vi "SetSettings.vi"(8 "error in (no error)":errorcluster, 10 "Variant":variant, 11 "NHRDCPower in":refnum<class "NHRDCPower.lvclass">) -> (0 "error out":errorcluster, 3 "NHRDCPower Out":refnum<class "NHRDCPower.lvclass">)   [LabVIEW 2018, in "AcPwrPlugins.lvlib" / "NHRDCPower.lvclass"]
doc: "This VI sets the configuration settings, measurement settings, and measurement refresh time."
uses:
  NHRDCPower.lvclass
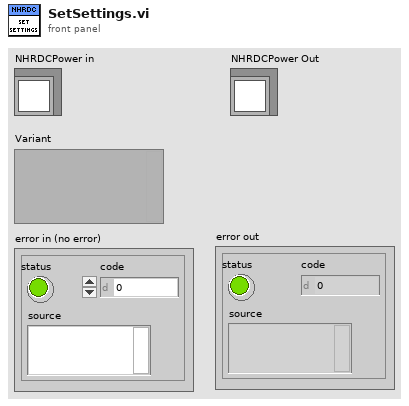
[diagram p1: front panel]
types:
  T1 = typedef "AcPwrPlugins.lvlib/NHRDCPower.lvclass/Device(s)Settings.ctl" = cluster{"MeasName":string, "Modules":T2}
  T2 = typedef "AcPwrPlugins.lvlib/NHRDCPower.lvclass/Modules.ctl" = cluster{"Handle":string, "Name":string, "id query (Yes)":bool, "reset device (Yes)":bool, "Connected":bool, "Initial Battery Detect Voltage (0)":dbl, "SafetySettings":cluster{"SetWatchDog?":bool, "Voltage (V)":dbl, "Current (A)":dbl, "Power (W)":dbl, "Voltage Delay (s)":dbl, "Current Delay (s)":dbl, "Power Delay (s)":dbl}, "Options String":string, "Aperture Time (s)":dbl, "operating state (Off)":i32, "OutputSettings":cluster{"Voltage (V)":dbl, "Current (A)":dbl, "Resistance (Ohms)":dbl, "Power (W)":dbl, "Enable Voltage":bool, "Enable Current":bool, "Enable Resistance":bool, "Enable Power":bool, "Macro After Step Delay  (s)":dbl, "Wait Value (V, A, W)":dbl, "Enable Wait":bool, "Wait on Value":i32}[], "SlewRate":cluster{"Set Voltage Rate V/S":dbl, "Set Current Rate A/S":dbl, "Set Resistance Rate R/S":dbl, "Set Power Rate W/S":dbl}, "Macro":cluster{"Save Macro?":bool, "Load Macro From File?":bool, "Run Macro Continuously?":bool, "Use Macros?":bool, "Load Macro File Path":string, "Save Macro File Path":string}, "Regulation Gain (1=100%)":dbl, "UpdatingOntheFly":bool}[]
  T3 = typedef "AcPwrPlugins.lvlib/NHRDCPower.lvclass/Measurements.ctl" = cluster{"Handle":string, "Name":string, "Enabled":bool, "Measurement Value":sgl, "Measurement Type":enum16{"Power", "Current", "Voltage"}}[]
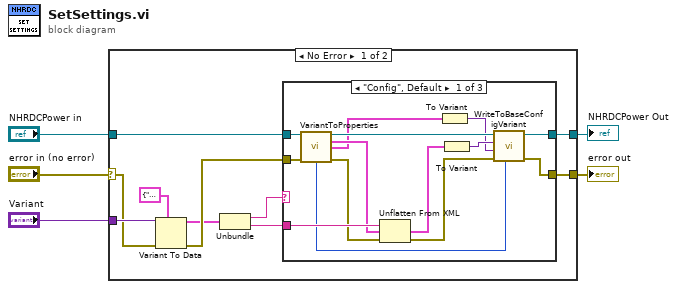
[diagram p0: block diagram]
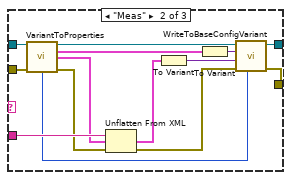
[diagram p2: hidden frame]
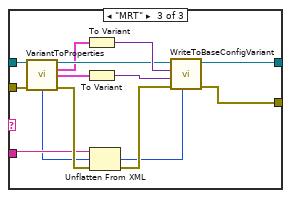
[diagram p3: hidden frame]
diagram:
  n1 = case shown="No Error" "error in (no error)" {
    selector: "error in (no error)" -> [w11 w59]
    tunnel: [w14 w59] -> w4
    tunnel: "NHRDCPower in" -> [w15 w58]
    tunnel: "Variant" -> [w12 _]
    tunnel: [w13 w58] -> w5
    frame No Error {
      n2 = Variant To Data(error in=w11, type=cluster{string, string} {"", ""}, Variant=w12) -> (data=w8:cluster{string, string}, error out=w9:errorcluster)
      n3 = Unbundle(w8) -> (w6:string, w7:string)
      n4 = case shown="\"Config\", Default" w6 {
        tunnel: [w21 w37 w52] -> w14
        tunnel: w15 -> [w28 w42 w57]
        tunnel: [w20 w36 w51] -> w13
        tunnel: w9 -> [w27 w41 w56]
        tunnel: w7 -> [w29 w43 w46]
        frame "Config", Default {
          n5 = call "VariantToProperties.vi"("NHRDCPower in"=w28, "error in (no error)"=w27) -> ("NHRDCPower out"=w19:refnum<class "NHRDCPower.lvclass">, "NHRDC"=w25:T1, "Meas"=w17:T3, "Measurement Refresh Time (ms)"=w18:u32, "error out"=w26:errorcluster)  [unwired: 7 in, 2 out]
          n6 = Unflatten From XML(xml string=w29, type=w25, error in (no error)=w26) -> (value=w24:T1, error out=w22:errorcluster)
          n7 = To Variant(anything=w17) -> (Variant=w16:variant)
          n8 = To Variant(anything=w24) -> (Variant=w23:variant)
          n9 = call "WriteToBaseConfigVariant.vi"("Measurement Refresh Time (ms)"=w18, "error in (no error)"=w22, "Meas"=w16, "Config"=w23, "NHRDCPower in"=w19) -> ("error out"=w21:errorcluster, "NHRDCPower out"=w20:refnum<class "NHRDCPower.lvclass">)  [unwired: 5 in]
        }
        frame "Meas" {
          n10 = call "VariantToProperties.vi"("NHRDCPower in"=w42, "error in (no error)"=w41) -> ("NHRDCPower out"=w35:refnum<class "NHRDCPower.lvclass">, "NHRDC"=w32:T1, "Meas"=w31:T3, "Measurement Refresh Time (ms)"=w34:u32, "error out"=w40:errorcluster)  [unwired: 7 in, 2 out]
          n11 = Unflatten From XML(xml string=w43, type=w31, error in (no error)=w40) -> (value=w30:T3, error out=w38:errorcluster)
          n12 = To Variant(anything=w30) -> (Variant=w33:variant)
          n13 = To Variant(anything=w32) -> (Variant=w39:variant)
          n14 = call "WriteToBaseConfigVariant.vi"("Measurement Refresh Time (ms)"=w34, "error in (no error)"=w38, "Meas"=w33, "Config"=w39, "NHRDCPower in"=w35) -> ("error out"=w37:errorcluster, "NHRDCPower out"=w36:refnum<class "NHRDCPower.lvclass">)  [unwired: 5 in]
        }
        frame "MRT" {
          n15 = call "VariantToProperties.vi"("NHRDCPower in"=w57, "error in (no error)"=w56) -> ("NHRDCPower out"=w50:refnum<class "NHRDCPower.lvclass">, "NHRDC"=w47:T1, "Meas"=w49:T3, "Measurement Refresh Time (ms)"=w45:u32, "error out"=w55:errorcluster)  [unwired: 7 in, 2 out]
          n16 = To Variant(anything=w47) -> (Variant=w54:variant)
          n17 = To Variant(anything=w49) -> (Variant=w48:variant)
          n18 = Unflatten From XML(xml string=w46, type=w45, error in (no error)=w55) -> (value=w44:u32, error out=w53:errorcluster)
          n19 = call "WriteToBaseConfigVariant.vi"("Measurement Refresh Time (ms)"=w44, "error in (no error)"=w53, "Meas"=w48, "Config"=w54, "NHRDCPower in"=w50) -> ("error out"=w52:errorcluster, "NHRDCPower out"=w51:refnum<class "NHRDCPower.lvclass">)  [unwired: 5 in]
        }
      }
    }
    frame Error {
    }
  }
  "error out" <- w4
  "NHRDCPower Out" <- w5
